vi "getSFP+testResult.vi"(10 "itemClusters":T1, 11 "itemName":string) -> (2 "sResult":string, 3 "result":bool)   [LabVIEW 2011]
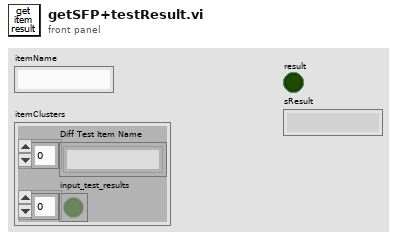
[diagram p1: front panel]
types:
  T1 = cluster{"Diff Test Item Name":string[], "input_test_results":bool[]}
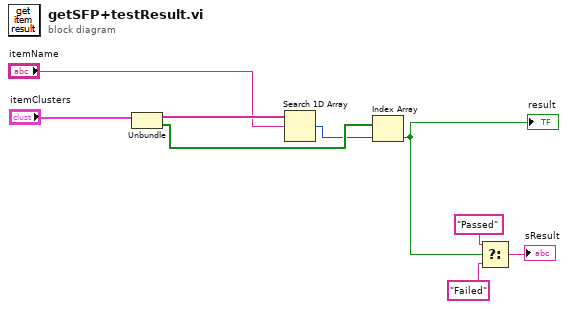
[diagram p0: block diagram]
diagram:
  n1 = Unbundle("itemClusters") -> ("Diff Test Item Name"=w8:string[], "input_test_results"=w6:bool[])
  n2 = Search 1D Array(1D array=w8, element="itemName") -> (index of element=w5:i32)  [unwired: 1 in]
  n3 = Index Array(array=w6, index=w5) -> (element=w2:bool)
  "result" <- w2
  n4 = Select(t="Passed", s=w2, f="Failed") -> (s? t:f=→"sResult":string)
